vi "Check Polygon Input.vi"(10 "Y In":dbl[](array[numeric]), 11 "X In":dbl[](array[numeric])) -> (0 "error":i32, 2 "Y Out":dbl[](array[numeric]), 3 "X Out":dbl[](array[numeric]))   [LabVIEW 2020, in "NI_AAL_Geometry.lvlib"]
uses:
  <vilib>/Analysis/NI_AAL_Geometry.lvlib
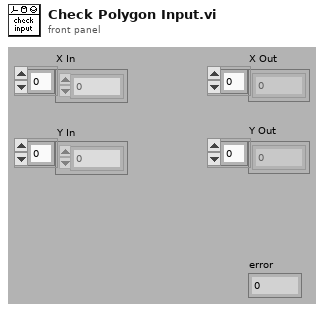
[diagram p1: front panel]
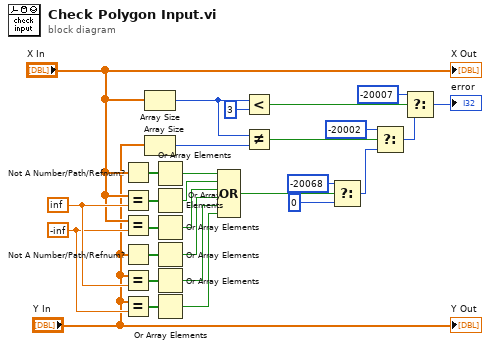
[diagram p0: block diagram]
diagram:
  w20 = -inf
  w21 = inf
  n1 = Not A Number/Path/Refnum?(number/path/refnum="X In") -> (NaN/Path/Refnum?=w19:bool[])
  n2 = Equal?(x="X In", y=w21) -> (x = y?=w18:bool[])
  n3 = Equal?(x="X In", y=w20) -> (x = y?=w17:bool[])
  n4 = Not A Number/Path/Refnum?(number/path/refnum="Y In") -> (NaN/Path/Refnum?=w16:bool[])
  n5 = Equal?(x="Y In", y=w21) -> (x = y?=w15:bool[])
  n6 = Equal?(x="Y In", y=w20) -> (x = y?=w14:bool[])
  n7 = Array Size(array="X In") -> (size(s)=w27:i32)
  n8 = Array Size(array="Y In") -> (size(s)=w29:i32)
  n9 = Or Array Elements(Boolean array=w19) -> (logical OR=w13:bool)
  n10 = Or Array Elements(Boolean array=w18) -> (logical OR=w12:bool)
  n11 = Or Array Elements(Boolean array=w17) -> (logical OR=w11:bool)
  n12 = Or Array Elements(Boolean array=w16) -> (logical OR=w10:bool)
  n13 = Or Array Elements(Boolean array=w15) -> (logical OR=w9:bool)
  n14 = Or Array Elements(Boolean array=w14) -> (logical OR=w8:bool)
  n15 = Compound Arithmetic op=OR(w13, w12, w11, w10, w9, w8) -> (w5:bool)
  n16 = Less?(x=w27, y=3) -> (x < y?=w4:bool)
  n17 = Not Equal?(x=w27, y=w29) -> (x != y?=w23:bool)
  n18 = Select(t=-20068, s=w5, f=0) -> (s? t:f=w22:i32)
  n19 = Select(t=-20002, s=w23, f=w22) -> (s? t:f=w28:i32)
  n20 = Select(t=-20007, s=w4, f=w28) -> (s? t:f=→"error":i32)
  "X Out" <- "X In"
  "Y Out" <- "Y In"
